vi "From Binary.vi"(6 "byte order":T1(ring), 8 "error in (no error)":errorcluster, 10 "Binary":string, 11 "Type in":refnum<class "Abs_String 1D.lvclass">) -> (0 "error out":errorcluster, 2 "Remaining":string, 3 "Type out":refnum<class "Abs_String 1D.lvclass">)   [LabVIEW 2021, in "Abs_String 1D.lvclass"]
uses:
  Abs_String 1D.lvclass
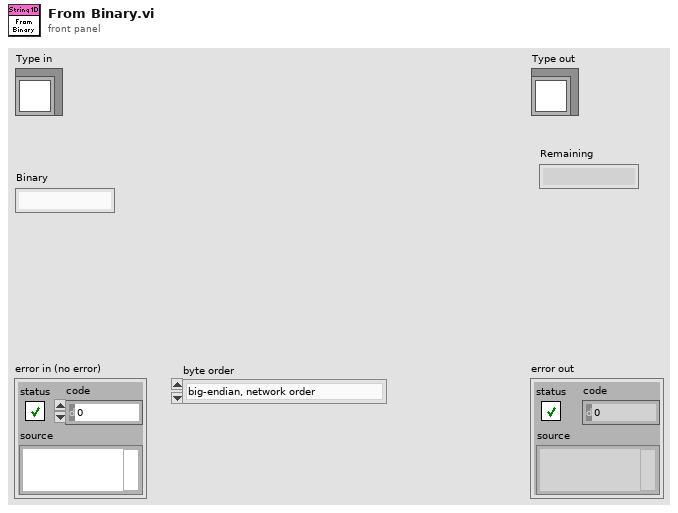
[diagram p1: front panel]
types:
  T1 = enum16{"big-endian, network order", "native, host order", "little-endian"}
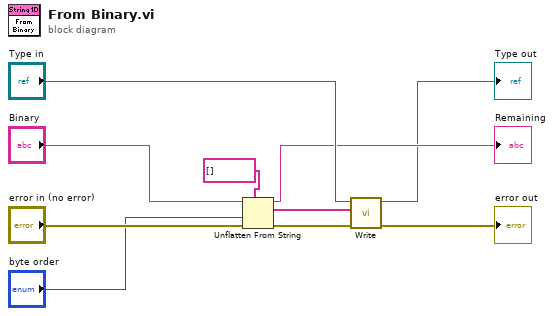
[diagram p0: block diagram]
diagram:
  n1 = Unflatten From String(type=string[] [], binary string="Binary", byte order (0:big-endian, network order)="byte order", error in (no error)="error in (no error)") -> (rest of the binary string=→"Remaining":string, value=w3:string[], error out=w2:errorcluster)  [unwired: 1 in]
  n2 = call-dynamic "Write.vi"("error in (no error)"=w2, "Array"=w3, "Abs_String in"="Type in") -> ("error out"=→"error out":errorcluster, "Abs_String out"=→"Type out":refnum<class "Abs_String 1D.lvclass">)  [unwired: 7 in]
